vi "remove channel from configuration.vi"(8 "error in":errorcluster, 10 "channel":refnum<class "TBM channel.lvclass">, 11 "sample module configuration in":refnum<class "sample module configuration.lvclass">) -> (0 "error out":errorcluster, 3 "sample module configuration out":refnum<class "sample module configuration.lvclass">)   [LabVIEW 2013, in "sample module configuration.lvclass"]
uses:
  sample module configuration.lvclass
  channel/TBM channel.lvclass
  sample module configuration.lvclass/sample module configuration.ctl
  <vilib>/NI/Tag Bus/tag/tag descriptor.lvclass/tag descriptor.ctl
  <vilib>/NI/Tag Bus/tag/tag descriptor.lvclass
  root configuration/TBM configuration.lvclass
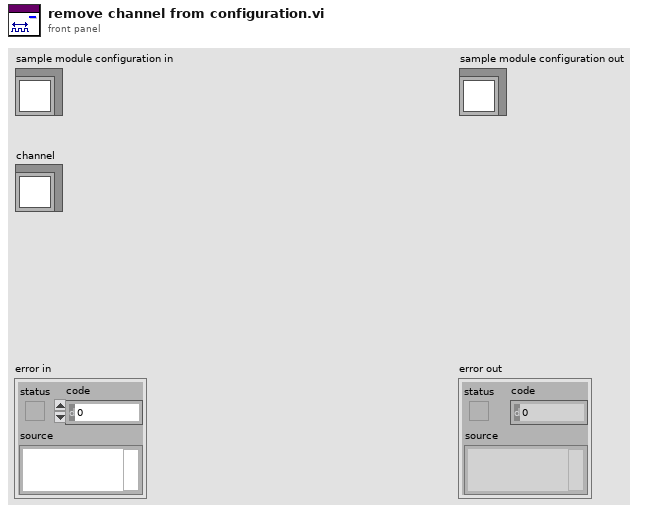
[diagram p1: front panel]
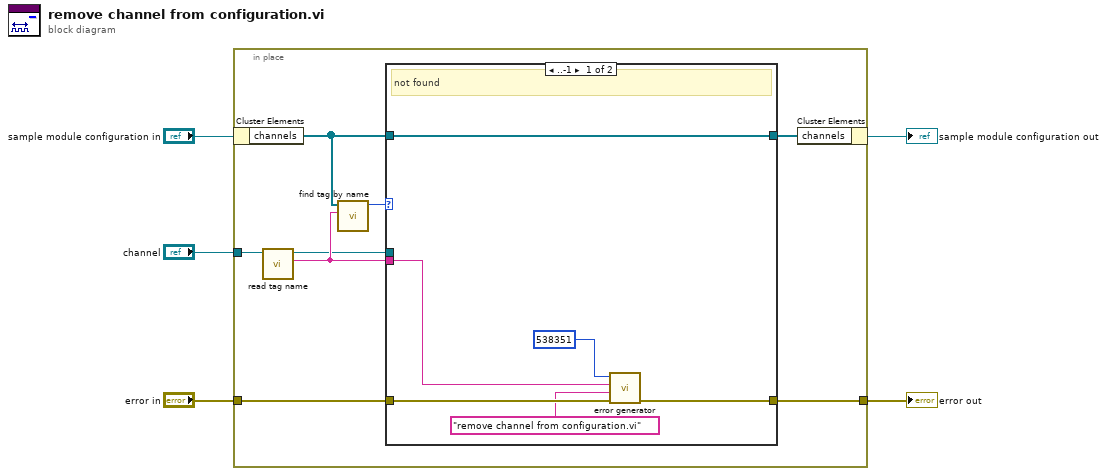
[diagram p0: block diagram]
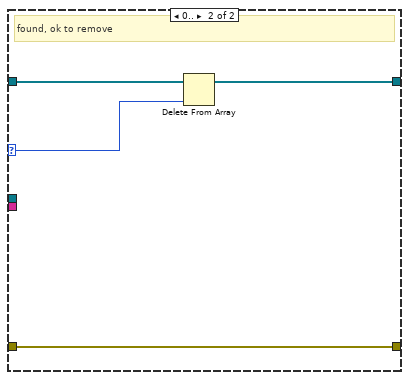
[diagram p2: hidden frame]
diagram:
  n1 = in-place {
    in-place-border: "channel" -> [w13]
    in-place-border: "error in" -> [w11]
    in-place-border: [w7] -> w1
    n2 = in-place-cluster #1("sample module configuration in") -> ("channels"=w8:refnum<class "TBM channel.lvclass">[])
    n3 = call <vilib>:"read tag name.vi"("system tag in"=w13) -> ("name"=w10:string, "system tag out"=w9:refnum<class "TBM channel.lvclass">)  [unwired: 8 in, 1 out]
    n4 = call <vilib>:"find tag by name.vi"("name"=w10, "tags in"=w8) -> ("index"=w12:i32)  [unwired: 9 in]
    n5 = case shown="..-1" w12 {
      selector: w12 -> [_ w20]
      tunnel: w11 -> [w19 w23]
      tunnel: w10 -> [w16 _]
      tunnel: w9 -> [_ _]
      tunnel: w8 -> [w15 w22]
      tunnel: [w18 w23] -> w7
      tunnel: [w15 w21] -> w6
      frame ..-1 {
        # "not found"
        n6 = call "error generator.vi"("error in"=w19, "source"="remove channel from configuration.vi", "append error message"=w16, "error code (0)"=538351) -> ("error out"=w18:errorcluster)  [unwired: 7 in]
      }
      frame 0.. {
        # "found, ok to remove"
        n7 = Delete From Array(array=w22, index=w20) -> (array with subset deleted=w21:refnum<class "TBM channel.lvclass">[])  [unwired: 1 in, 1 out]
      }
    }
    n8 = in-place-cluster #1("channels"=w6) -> (→"sample module configuration out":refnum<class "sample module configuration.lvclass">)
  }
  "error out" <- w1
